vi "Sort_Insect-data-array_Length.vi"(1 "Insect-data-array":dbl[][](array[numeric])) -> (0 "Insect-data-array (sorted-length)":dbl[][](array[numeric]))   [LabVIEW 2024]
doc: "Sorts the insect-data-array based on insect length with largest insects first"
uses:
  1b2f16e1-6f8a-40ae-96ac-6b9022457792.vi
  <vilib>/Array/Sort 2D Array - Pop Stack.vi
  <vilib>/Array/Sort 2D Array - Push Stack.vi
  1b2f16e1-6f8a-40ae-96ac-6b9022457792.vi/269d4b3b-47f5-49e3-8884-44851e4dd9d5.vi
  1b2f16e1-6f8a-40ae-96ac-6b9022457792.vi/6d99389c-673d-4efb-bf33-19b32bcf4cf8.vi
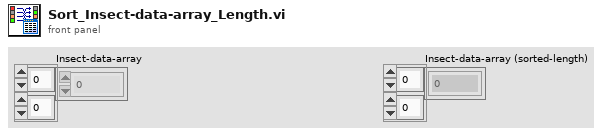
[diagram p1: front panel]
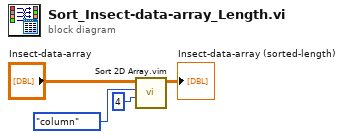
[diagram p0: block diagram]
diagram:
  n1 = call "Sort 2D Array.vim"("index"=4, "dimension to index (column)"=enum16{"column", "row"}."column", "2D array"="Insect-data-array") -> ("sorted 2D array"=→"Insect-data-array (sorted-length)":dbl[][])  [unwired: 7 in, 1 out]
